vi "Build Waveform Channels.vi"(8 "error in (no error)":errorcluster, 11 "Injector section ref in":T1 format="%.0x") -> (0 "error out":errorcluster, 2 "Waveform channel array out":T2[](array[typedef]), 3 "Injector section ref out":T1 format="%.0x")   [LabVIEW 2019, in "Fuel Injector Analysis Addon System Explorer.lvlib"]
uses:
  Fuel Injector Analysis Addon System Explorer.lvlib
  <vilib>/NI VeriStand/Custom Device API/Custom Device Item Ref.ctl
  <vilib>/NI VeriStand/Custom Device API/Waveform Data Reference.ctl
  Addon Shared/SubVIs/Constants.vi
  <vilib>/NI VeriStand/Custom Device Tools/Custom Device Utility Library/NI VeriStand - Search for Item by GUID.vi
  <vilib>/NI VeriStand/Custom Device Tools/Custom Device Utility Library/Custom Device Utility Library.lvlib
  Addon Shared/Fuel Injector Analysis Addon Shared.lvlib
  <vilib>/NI VeriStand/Custom Device API/Custom Device API.lvlib
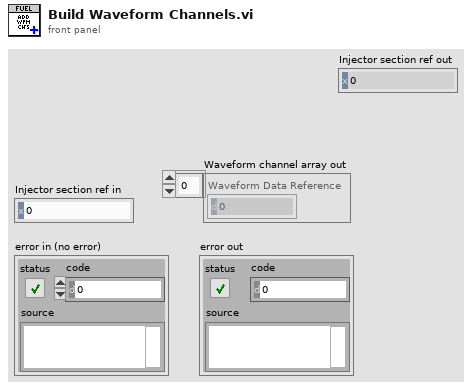
[diagram p1: front panel]
types:
  T1 = typedef "Custom Device API.lvlib/Custom Device Item Ref.ctl" = u64
  T2 = typedef "Custom Device API.lvlib/Waveform Data Reference.ctl" = i32
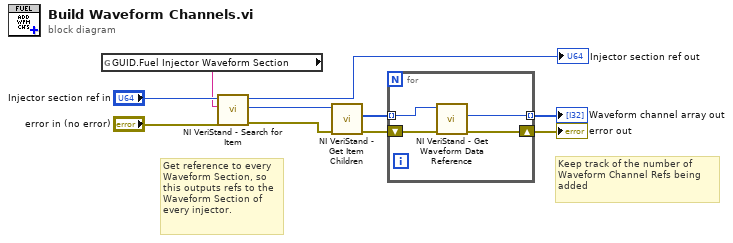
[diagram p0: block diagram]
diagram:
  # "Keep track of the number of\nWaveform Channel Refs being\nadded"
  # "Get reference to every\nWaveform Section, so\nthis outputs refs to the\nWaveform Section of \nevery injector."
  n1 = global read "Constants.vi" "GUID.Fuel Injector Waveform Section"() -> (w5:string)
  n2 = call-poly <vilib>:"NI VeriStand - Search for Item.vi"("error in"="error in (no error)", "Item GUID"=w5, "Section Ref in"="Injector section ref in") -> ("error out"=w7:errorcluster, "Item Ref"=w6:T1, "Section Ref out"=→"Injector section ref out":T1)  [unwired: 5 in, 1 out]
  n3 = call <vilib>:"NI VeriStand - Get Item Children.vi"("error in (no error)"=w7, "Item Ref in"=w6) -> ("error out"=w3:errorcluster, "Child Refs"=w2:T1[])  [unwired: 6 in, 2 out]
  n4 = for {
    tunnel: w2 -> [w14] mode=indexing
    shift-right: [w12] -> w8
    shift-left: w3 -> [w13]
    tunnel: [w11] -> w4 mode=indexing
    n5 = call <vilib>:"NI VeriStand - Get Waveform Data Reference.vi"("error in (no error)"=w13, "Waveform Ref in"=w14) -> ("error out"=w12:errorcluster, "Waveform Data Reference"=w11:T2)  [unwired: 7 in, 1 out]
  }
  "error out" <- w8
  "Waveform channel array out" <- w4
